vi "Artiq Client Delete.vi"(0 "Kasli Wrapper in":refnum<class "Kasli Wrapper 2.0.lvclass">, 11 "error in (no error)":errorcluster) -> (4 "Kasli Wrapper out":refnum<class "Kasli Wrapper 2.0.lvclass">, 6 "standard output":string, 8 "standard error":string, 10 "return code":i32, 15 "error out":errorcluster)   [LabVIEW 2020, in "Kasli Wrapper 2.0.lvlib" / "Kasli Wrapper 2.0.lvclass"]
doc: "This VI is used to submit (i.e. enqueue) a new ARTIQ script into the pipeline of the Master.\nIf the Dummy flag is set to True, the script is submitted with the artiq_run command, ignoring the connection with a master.\nDAQ flag is used for specifying if the connection with the DAQ should be established by the script or is done outside."
uses:
  Kasli Wrapper 2.0.lvclass
  Ancestor/Ancestor/Ancestor.lvclass/Ancestor.ctl
  FGV/Error Memory/Get Error Description.vi
  Support VIs/Get PC name.vi
  Ancestor/Ancestor/Read ID.vi
  Support VIs/Get Class Name.vi
  FGV/Error Memory/Error Memory Core.vi
  <vilib>/AdvancedString/Delimited String to 1D String Array.vi
  Support VIs/Circus Root Path.vi
  FGV/Error Memory/Error Crt Lvl checker.vi
  FGV/Error Memory/Error Memory Core.vi/40c8088d-b597-4017-91af-faa98e00292e.vi
  FGV/Error Memory/Error Memory Core.vi/d4a3ab98-063c-4e44-b43d-fbdcfe6c2be2.vi
  Support VIs/Global Memory.vi
  <vilib>/Utility/LVClass/Get LV Class Name.vi
  Support VIs/Is in Packed Library.vi
  Support VIs/TALOS Root path.vi
  Support VIs/Read CSV worksheet.vi
  Support VIs/Global Constants.vi
  <vilib>/Utility/error.llb/General Error Handler.vi
  Ancestor/Ancestor/Ancestor.lvclass
  <vilib>/Comparison/Equal/Equal Functor/Equal Functor.lvclass
  TALOS.lvlib
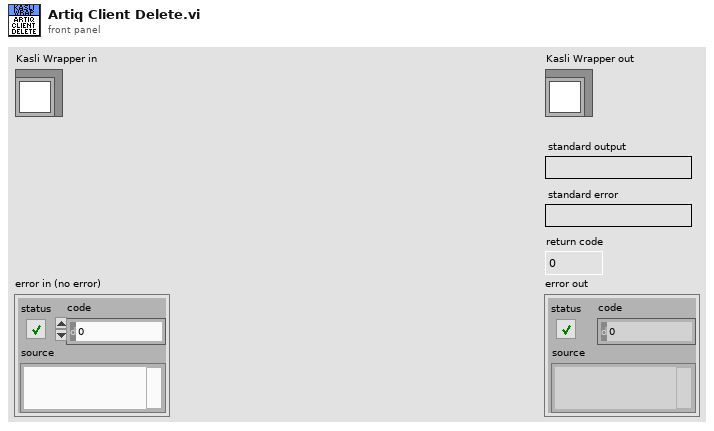
[diagram p1: front panel]
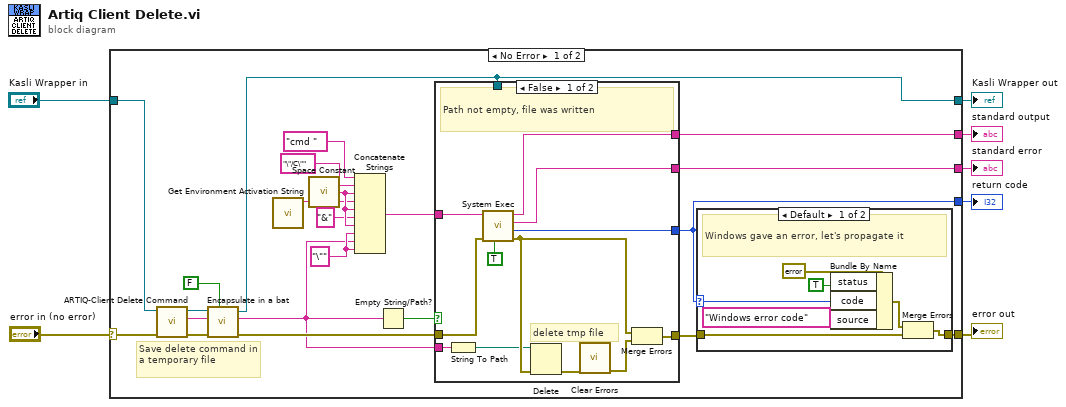
[diagram p0: block diagram]
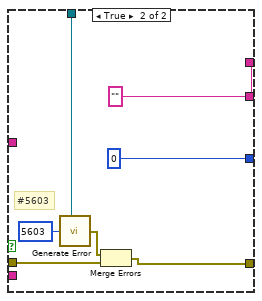
[diagram p3: hidden frame]
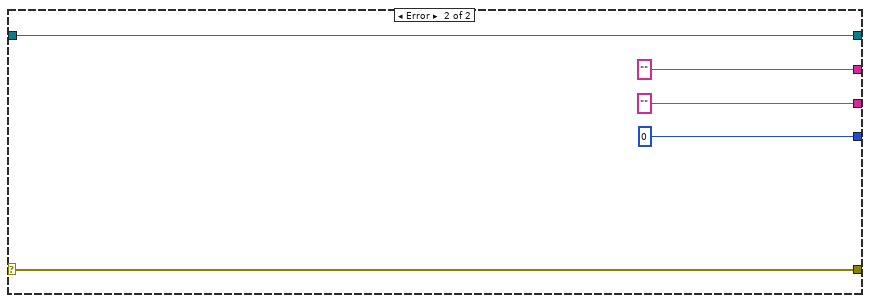
[diagram p4: hidden frame]
diagram:
  n1 = case shown="No Error" "error in (no error)" {
    selector: "error in (no error)" -> [w13 w61]
    tunnel: [w24 w61] -> w6
    tunnel: "Kasli Wrapper in" -> [w14 w60]
    tunnel: [w15 w60] -> w4
    tunnel: [w17 "" ("standard output")] -> w1
    tunnel: [w29 "" ("standard error")] -> w2
    tunnel: [w16 0 ("return code")] -> w3
    frame No Error {
      w22 = "\"" ("string")
      # "Save delete command in a temporary file"
      n2 = call-dynamic "ARTIQ-Client Delete Command.vi"("error in (no error)"=w13, "Kasli Wrapper 2.0 in"=w14) -> ("error out"=w10:errorcluster, "artiq-client delete"=w12:string, "Kasli Wrapper 2.0 out"=w11:refnum<class "Kasli Wrapper 2.0.lvclass">)  [unwired: 7 in]
      n3 = call-dynamic "Encapsulate in a bat.vi"("Overwrite?"=FALSE, "error in (no error)"=w10, "command"=w12, "Kasli Wrapper in"=w11) -> ("error out"=w28:errorcluster, "bat out"=w8:string, "Kasli Wrapper out"=w15:refnum<class "Kasli Wrapper 2.0.lvclass">)  [unwired: 5 in]
      n4 = call "Get Environment Activation String.vi"() -> ("Conda Activation String"=w18:string)  [unwired: 10 in, 1 out]
      n5 = call <vilib>:"Space Constant.vi"() -> ("String"=w23:string)
      n6 = Concatenate Strings("cmd " ("command line"), "\"/C\"", w23, w18, w23, "&" ("string"), w23, w22, w8, w22) -> (w26:string)
      n7 = Empty String/Path?(string/path=w8) -> (empty?=w27:bool)
      n8 = case shown="False" w27 {
        tunnel: w26 -> [w47 _]
        tunnel: [w39 w50] -> w25
        tunnel: [w46 w56] -> w17
        tunnel: [w45 w56] -> w29
        tunnel: [w44 0 ("return code")] -> w16
        tunnel: w28 -> [w43 w52]
        tunnel: w15 -> [_ w54]
        tunnel: w8 -> [w42 _]
        frame False {
          # "delete tmp file"
          # "Path not empty, file was written"
          n9 = String To Path(string=w42) -> (path=w41:path)
          n10 = call <vilib>:"System Exec.vi"("run minimized? (F)"=TRUE, "error in (no error)"=w43, "command line"=w47) -> ("error out"=w49:errorcluster, "return code"=w44:i32, "standard error"=w45:string, "standard output"=w46:string)  [unwired: 5 in]
          n11 = Delete(path (use dialog)=w41, error in=w49) -> (error out=w40:errorcluster)  [unwired: 3 in, 2 out]
          n12 = call <vilib>:"Clear Errors.vi"("error in (no error)"=w40) -> ("error out"=w38:errorcluster)  [unwired: 5 in, 1 out]
          n13 = Merge Errors(w49, w38) -> (w39:errorcluster)
        }
        frame True {
          w56 = "" ("standard output")
          # "#5603"
          n14 = call "Generate Error.vi"("Class"=w54, "Error Code"=5603) -> ("error out"=w51:errorcluster)  [unwired: 5 in]
          n15 = Merge Errors(w51, w52) -> (w50:errorcluster)
        }
      }
      n16 = case shown="Default" w16 {
        selector: w16 -> [w35 _]
        tunnel: w25 -> [w32 w37]
        tunnel: [w31 w37] -> w24
        frame Default {
          # "Windows gave an error, let's propagate it"
          n17 = Bundle By Name(cluster=errorcluster {"status"=FALSE, "code"=0, "source"=""} ("error constant"), "status"=TRUE, "code"=w35, "source"="Windows error code") -> (w33:errorcluster)
          n18 = Merge Errors(w33, w32) -> (w31:errorcluster)
        }
        frame 0 {
          # "Error code is OK"
        }
      }
    }
    frame Error {
    }
  }
  "Kasli Wrapper out" <- w4
  "error out" <- w6
  "return code" <- w3
  "standard error" <- w2
  "standard output" <- w1
